vi "Set User Password.vi"(0 "iUser Configuration Manager DVR":refnum<data-value>, 5 "Username":string, 7 "Current Password":string, 9 "New Password":string, 11 "error in":errorcluster) -> (4 "dup iUser Configuration Manager DVR":refnum<data-value>, 6 "Found":bool, 15 "error out":errorcluster)   [LabVIEW 2019, in "User Configuration Manager.lvlib" / "By Ref.lvlib"]
doc: "Sets the password of the user specified by user name."
uses:
  <vilib>/gpm_packages/@cs/user-manager/Source/User Configuration Manager Ref/By Ref.lvlib
  <vilib>/gpm_packages/@cs/user-manager/Source/iUser Configuration Manager/iUser Configuration Manager.lvclass
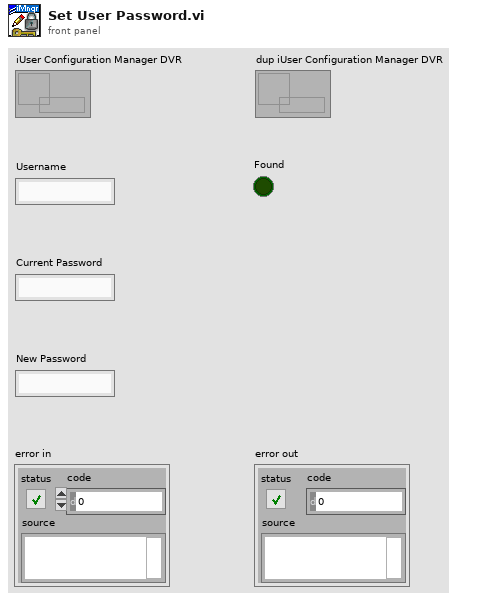
[diagram p1: front panel]
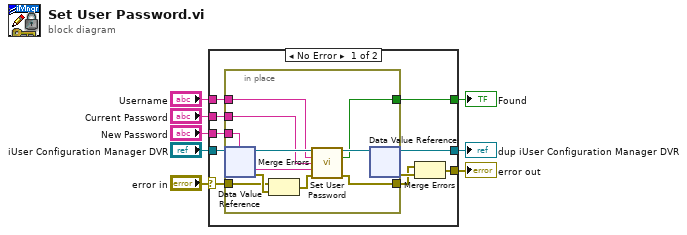
[diagram p0: block diagram]
diagram:
  n1 = case shown="No Error" "error in" {
    selector: "error in" -> [w16 w30]
    tunnel: "iUser Configuration Manager DVR" -> [w18 w29]
    tunnel: [w17 w30] -> w7
    tunnel: [w13 w29] -> w5
    tunnel: "Username" -> [w12 _]
    tunnel: "Current Password" -> [w11 _]
    tunnel: "New Password" -> [w10 _]
    tunnel: [w9 _] -> w1
    frame No Error {
      n2 = in-place "IPES" {
        in-place-border: [w23] -> w14
        in-place-border: w16 -> [w27]
        in-place-border: w12 -> [w22]
        in-place-border: w11 -> [w19]
        in-place-border: w10 -> [w21]
        in-place-border: [w24] -> w9
        n3 = in-place-dvr #1(w18) -> (w26:refnum<class "iUser Configuration Manager.lvclass">, w28:errorcluster)
        n4 = Merge Errors(w27, w28) -> (w20:errorcluster)
        n5 = call-dynamic "Set User Password.vi"("iUser Configuration Manager in"=w26, "Username"=w22, "Current Password"=w19, "New Password"=w21, "error in (no error)"=w20) -> ("iUser Configuration Manager out"=w25:refnum<class "iUser Configuration Manager.lvclass">, "Found"=w24:bool, "error out"=w23:errorcluster)  [unwired: 8 in]
        n6 = in-place-dvr #1(w25) -> (w13:refnum<data-value>, w15:errorcluster)
      }
      n7 = Merge Errors(w14, w15) -> (w17:errorcluster)
    }
    frame Error {
    }
  }
  "error out" <- w7
  "dup iUser Configuration Manager DVR" <- w5
  "Found" <- w1
